vi "vector_v1.vi"() -> ()   [LabVIEW 2009]
panel:
  in  "stop":bool
  in  "Slide":u8(slide)=4 scale=0.0..7.0
  out "LED-ul selectat":bool
  in  "Vector LED-uri":bool[](array[boolean])=[TRUE, FALSE, TRUE, TRUE, FALSE, FALSE, FALSE, TRUE]
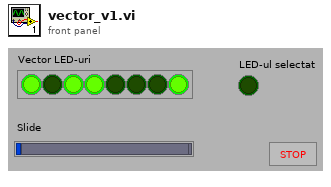
[diagram p1: front panel]
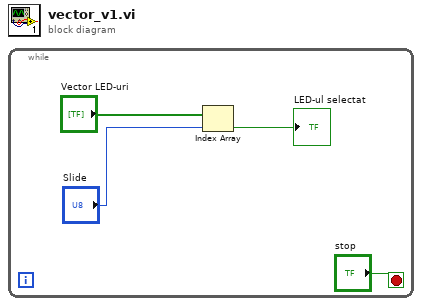
[diagram p0: block diagram]
diagram:
  n1 = while {
    stop <- "stop" stop-if-true
    n2 = Index Array(array="Vector LED-uri", index="Slide") -> (element=→"LED-ul selectat":bool)
  }
